vi "Write Header - Preamp Gain.vi"(8 "error in (no error)":errorcluster, 11 "Save Image in":refnum<class "Save Image.lvclass">) -> (0 "error out":errorcluster, 3 "Save Image out":refnum<class "Save Image.lvclass">)   [LabVIEW 2018, in "Save Image.lvclass"]
uses:
  Save Image.lvclass
  <vilib>/Utility/file.llb/Read Delimited Spreadsheet (string).vi
  Simulated_Header/Simulated_Header.lvclass
  Simulated_Header/write keyword - float.vi
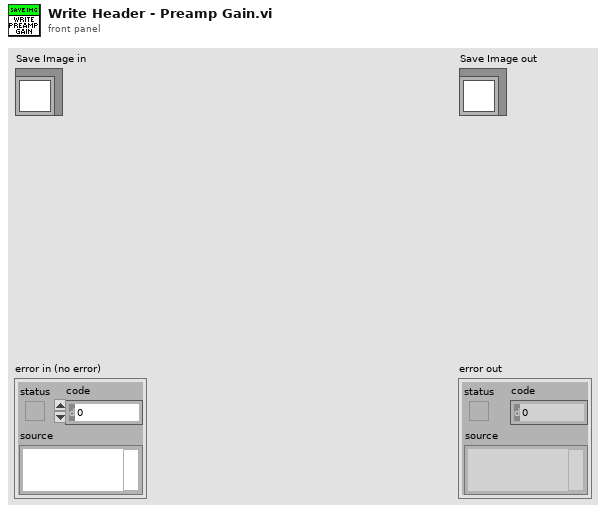
[diagram p1: front panel]
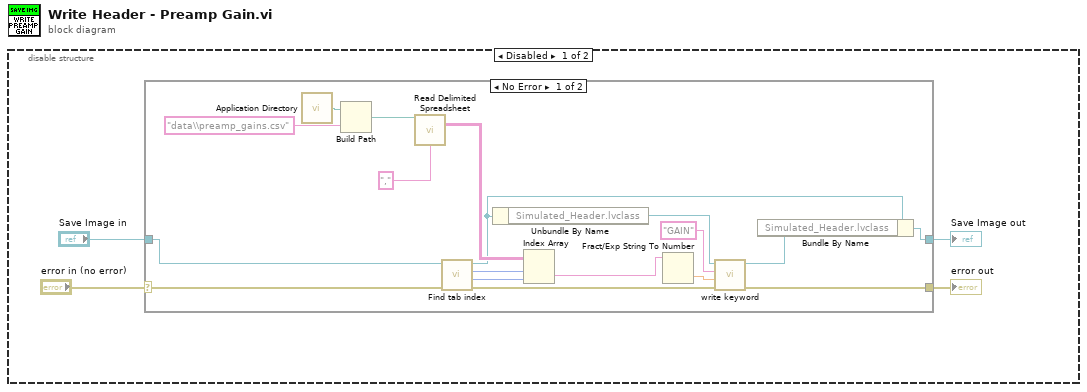
[diagram p0: block diagram]
diagram:
  n1 = disable-structure shown="Disabled" {
    frame Disabled {
      n2 = case shown="No Error" "error in (no error)" {
        selector: "error in (no error)" -> [w15 w24]
        tunnel: [w8 w24] -> w3
        tunnel: [w11 w23] -> w1
        tunnel: "Save Image in" -> [w16 w23]
        frame No Error {
          n3 = call <vilib>:"Application Directory.vi"() -> ("Application Directory"=w20:path)
          n4 = Build Path(base path=w20, name or relative path="data\\preamp_gains.csv") -> (appended path=w19:path)
          n5 = call-poly <vilib>:"Read Delimited Spreadsheet.vi"("file path (dialog if empty)"=w19, "delimiter (\\t)"="," ("delimiter (\\t)")) -> ("all rows"=w18:string[][])  [unwired: 8 in, 5 out]
          n6 = call "Find tab index.vi"("error in (no error)"=w15, "Save Image in"=w16) -> ("error out"=w7:errorcluster, "column"=w13:i32, "row"=w14:i32, "Save Image out"=w12:refnum<class "Save Image.lvclass">)  [unwired: 6 in]
          n7 = Unbundle By Name(w12) -> ("Simulated_Header.lvclass"=w10:refnum<class "Simulated_Header.lvclass">)
          n8 = Index Array(array=w18, index (row)=w14, index (col)=w13) -> (element=w17:string)
          n9 = Fract/Exp String To Number(string=w17) -> (number=w6:dbl)  [unwired: 3 in, 1 out]
          n10 = call-poly "write keyword.vi"("error in (no error)"=w7, "Value"=w6, "keyword"="GAIN", "Simulated_Header in"=w10) -> ("error out"=w8:errorcluster, "Simulated_Header out"=w9:refnum<class "Simulated_Header.lvclass">)  [unwired: 6 in]
          n11 = Bundle By Name(cluster=w12, "Simulated_Header.lvclass"=w9) -> (w11:refnum<class "Save Image.lvclass">)
        }
        frame Error {
        }
      }
      "error out" <- w3
      "Save Image out" <- w1
    }
    frame Enabled {
    }
  }
